vi "Insight_Valid_Vector_Clock_Transform.vi"(8 "error in (no error)":errorcluster, 9 "Input Valid Vector":i32[](array[numeric]), 10 "Laser Drive Clk":i32, 11 "Data Sample Clk":i32) -> (0 "error out":errorcluster, 1 "Output Valid Vector":i32[](array[numeric]))   [LabVIEW 2024]
doc: "Insight Photonic Solutions\n\nThis transforms the Data Valid Vector from the indices prescribed by the laser's Drive Clock, to the indices determined by the Data Sampling Clock. For example, the laser Drive Clock may be 400MHz, but the sample clock could be 800MHz.\n\nRecommended Implementation: Call this VI when a new acquisition clock rate is set, and at the set-up of an acquisition sequence. The Valid Vector transformation only needs to be performed once, for a given sweep calibration and acquisition clock rate.\n\nINPUTS\nData Sample Clock - the clock rate, in MHz, used to sample the data.\nLaser Drive Clock - the clock rate, in MHz, the laser sweeps. Default is 400MHz.\nInput Valid Vector - The Data Valid Vector (DVV) generated from the laser's Data Invalid Vector that corresponds to the laser's Drive Clock rate.\n\nOUTPUT\nOutput Valid Vector - The Data Valid Vector re-scaled to the Data Sample Clock rate. Use the Output DVV to remove hold points from the raw data measured at the Data Sample Clock rate.\n\nver 1.0 - original release\n\nCopyright 2014"
uses:
  <vilib>/Analysis/NI_AALPro.lvlib
panel:
  out "DVV Time Check":cluster{dbl[], dbl[]}[](graph)
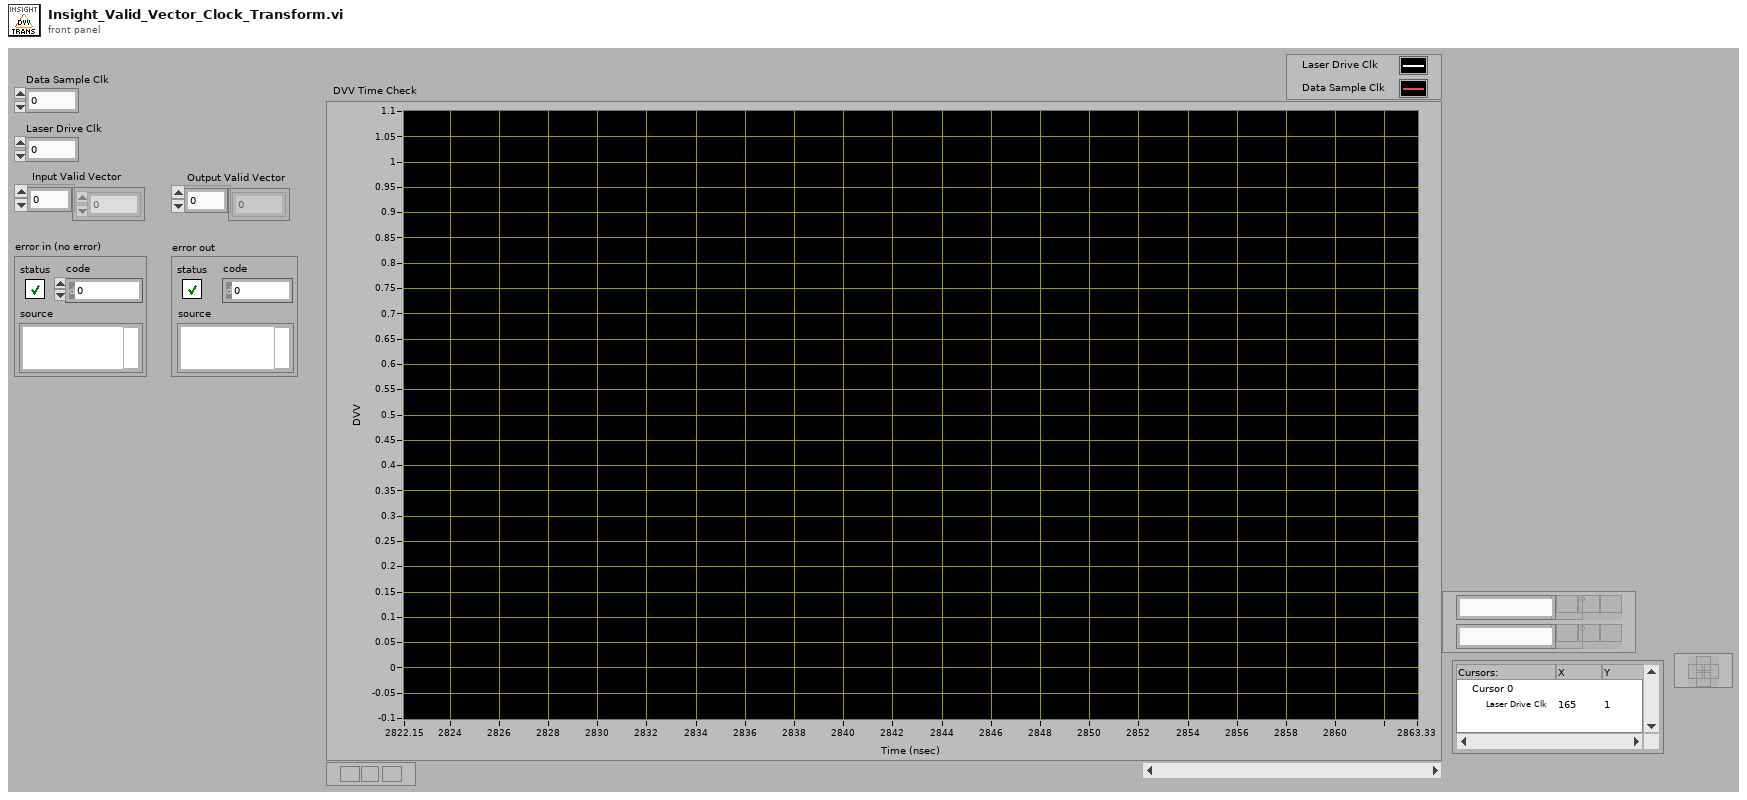
[diagram p1: front panel]
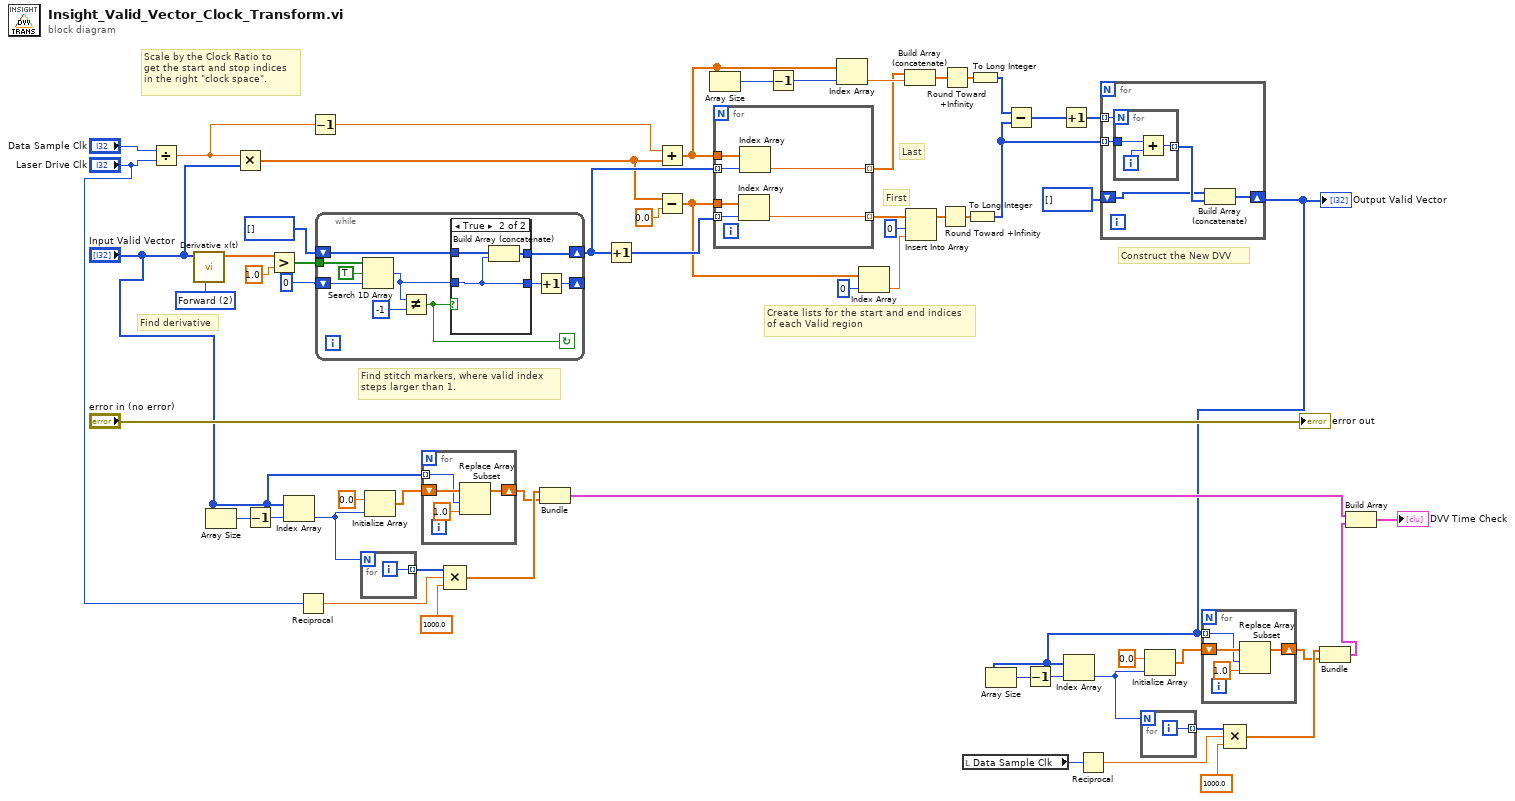
[diagram p0: block diagram]
diagram:
  w58 = u16 2 items=["2nd Order Central", "4th Order Central", "Forward", "Backward"] ("method")
  # "Scale by the Clock Ratio to\nget the start and stop indices \nin the right \"clock space\"."
  # "Construct the New DVV"
  # "Create lists for the start and end indices\nof each Valid region"
  # "First"
  # "Last"
  # "Find stitch markers, where valid index\nsteps larger than 1."
  # "Find derivative"
  n1 = Divide(x="Data Sample Clk", y="Laser Drive Clk") -> (x/y=w16:dbl)
  n2 = call <vilib>:"Derivative x(t).vi"("method"=w58, "X"="Input Valid Vector") -> ("dX/dt"=w49:dbl[])  [unwired: 8 in, 1 out]
  n3 = Array Size(array="Input Valid Vector") -> (size(s)=w46:i32)
  n4 = Multiply(x=w16, y="Input Valid Vector") -> (x*y=w14:dbl[])
  n5 = Decrement(x=w46) -> (x-1=w47:i32)
  n6 = Greater?(x=w49, y=1.0) -> (0:w56:bool[])
  n7 = Index Array(array="Input Valid Vector", index=w47) -> (element=w44:i32)
  n8 = Reciprocal(x="Laser Drive Clk") -> (1/x=w41:dbl)
  n9 = Decrement(x=w16) -> (x-1=w15:dbl)
  n10 = while {
    tunnel: w56 -> [w70]
    shift-right: [w61] -> _
    shift-left: 0 -> [w66]
    shift-right: [w63] -> w17
    shift-left: i32[] [] -> [w62]
    stop <- w64 continue-if-true
    n11 = Search 1D Array(1D array=w70, element=TRUE, start index (0)=w66) -> (index of element=w67:i32)
    n12 = Not Equal?(x=w67, y=-1) -> (x != y?=w64:bool)
    n13 = case shown="True" w64 {
      tunnel: w67 -> [w71 w73]
      tunnel: [w71 w73] -> w65
      tunnel: [w72 w75] -> w63
      tunnel: w62 -> [w72 w74]
      frame False {
      }
      frame True {
        n14 = Build Array (concatenate)(w74, w73) -> (w75:i32[])
      }
    }
    n15 = Increment(x=w65) -> (x+1=w61:i32)
  }
  n16 = for {
    N: w44 -> [_]
    tunnel: [w76] -> w43 mode=indexing
    i -> [w76]
  }
  n17 = Initialize Array(0.0 ("element"), w44) -> (w39:dbl[])
  n18 = for {
    tunnel: "Input Valid Vector" -> [w78] mode=indexing
    shift-right: [w77] -> w36
    shift-left: w39 -> [w80]
    n19 = Replace Array Subset(array=w80, new element=1.0 ("new element/subarray"), index=w78) -> (w77:dbl[])
  }
  n20 = Compound Arithmetic op=MULTIPLY(w43, w41, 1000.0 ("value")) -> (w37:dbl[])
  n21 = Bundle(w37, w36) -> (w24:cluster{dbl[], dbl[]})  [unwired: 1 in]
  n22 = Increment(x=w17) -> (x+1=w18:i32[])
  n23 = Add(x=w15, y=w14) -> (x+y=w12:dbl[])
  n24 = Subtract(x=w14, y=0.0) -> (x-y=w13:dbl[])
  n25 = Array Size(array=w12) -> (size(s)=w52:i32)
  n26 = for {
    tunnel: w12 -> [w86]
    tunnel: w17 -> [w85] mode=indexing
    tunnel: w18 -> [w84] mode=indexing
    tunnel: [w81] -> w6 mode=indexing
    tunnel: [w82] -> w9 mode=indexing
    tunnel: w13 -> [w83]
    n27 = Index Array(array=w83, index=w84) -> (element=w81:dbl)
    n28 = Index Array(array=w86, index=w85) -> (element=w82:dbl)
  }
  n29 = Decrement(x=w52) -> (x-1=w48:i32)
  n30 = Index Array(array=w12, index=w48) -> (element=w10:dbl)
  n31 = Index Array(array=w13, index=0) -> (element=w5:dbl)
  n32 = Build Array (concatenate)(w9, w10) -> (w8:dbl[])
  n33 = Insert Into Array(array=w6, index=0 ("new element/subarray"), new element=w5) -> (w3:dbl[])
  n34 = Round Toward +Infinity(x=w3) -> (ceil(x): smallest int >= x=w2:dbl[])
  n35 = Round Toward +Infinity(x=w8) -> (ceil(x): smallest int >= x=w7:dbl[])
  n36 = local read "Data Sample Clk"() -> (w25:i32)
  n37 = To Long Integer(number=w2) -> (32bit integer=w4:i32[])
  n38 = To Long Integer(number=w7) -> (32bit integer=w11:i32[])
  n39 = Subtract(x=w11, y=w4) -> (x-y=w19:i32[])
  n40 = Increment(x=w19) -> (x+1=w20:i32[])
  n41 = Reciprocal(x=w25) -> (1/x=w30:dbl)
  n42 = for {
    tunnel: w20 -> [w91] mode=indexing
    tunnel: w4 -> [w90] mode=indexing
    shift-right: [w89] -> w21
    shift-left: i32[] [] -> [w87]
    n43 = for {
      N: w91 -> [_]
      tunnel: w90 -> [w93]
      tunnel: [w92] -> w88 mode=indexing
      i -> [w94]
      n44 = Add(x=w93, y=w94) -> (x+y=w92:i32)
    }
    n45 = Build Array (concatenate)(w87, w88) -> (w89:i32[])
  }
  "Output Valid Vector" <- w21
  n46 = Array Size(array=w21) -> (size(s)=w34:i32)
  n47 = Decrement(x=w34) -> (x-1=w35:i32)
  n48 = Index Array(array=w21, index=w35) -> (element=w32:i32)
  n49 = for {
    N: w32 -> [_]
    tunnel: [w95] -> w31 mode=indexing
    i -> [w95]
  }
  n50 = Initialize Array(0.0 ("element"), w32) -> (w28:dbl[])
  n51 = for {
    tunnel: w21 -> [w97] mode=indexing
    shift-right: [w96] -> w26
    shift-left: w28 -> [w99]
    n52 = Replace Array Subset(array=w99, new element=1.0 ("new element/subarray"), index=w97) -> (w96:dbl[])
  }
  n53 = Compound Arithmetic op=MULTIPLY(w31, w30, 1000.0 ("value")) -> (w27:dbl[])
  n54 = Bundle(w27, w26) -> (w23:cluster{dbl[], dbl[]})  [unwired: 1 in]
  n55 = Build Array(w24, w23) -> (→"DVV Time Check":cluster{dbl[], dbl[]}[])
  "error out" <- "error in (no error)"
